vi "Autonomous Independent.vi"   [LabVIEW 2019]
doc: "This VI is called when autonomous begins, and will automatically be terminated when autonomous ends. You can carry out timed or sensor driven robot movement independently without needing to return to the caller."
uses:
  Robot Global Data.vi
  <vilib>/Rock Robotics/Network Tables/NT Read Number.vi
  <vilib>/Rock Robotics/Network Tables/NT Read String.vi
  <vilib>/Rock Robotics/Network Tables/NT Write Numeric Array.vi
panel:
  # "Be sure to right-click and choose Data Operations>>Make Current Value default if you want to save the array values with the VI"
types:
  T1 = typedef "WPI_JoystickDevRef.ctl" = cluster{"Device":T2}
  T2 = typedef "WPI_JoystickDeviceEnum.ctl" = enum16{"USB 0", "USB 1", "USB 2", "USB 3", "USB 4", "USB 5"}
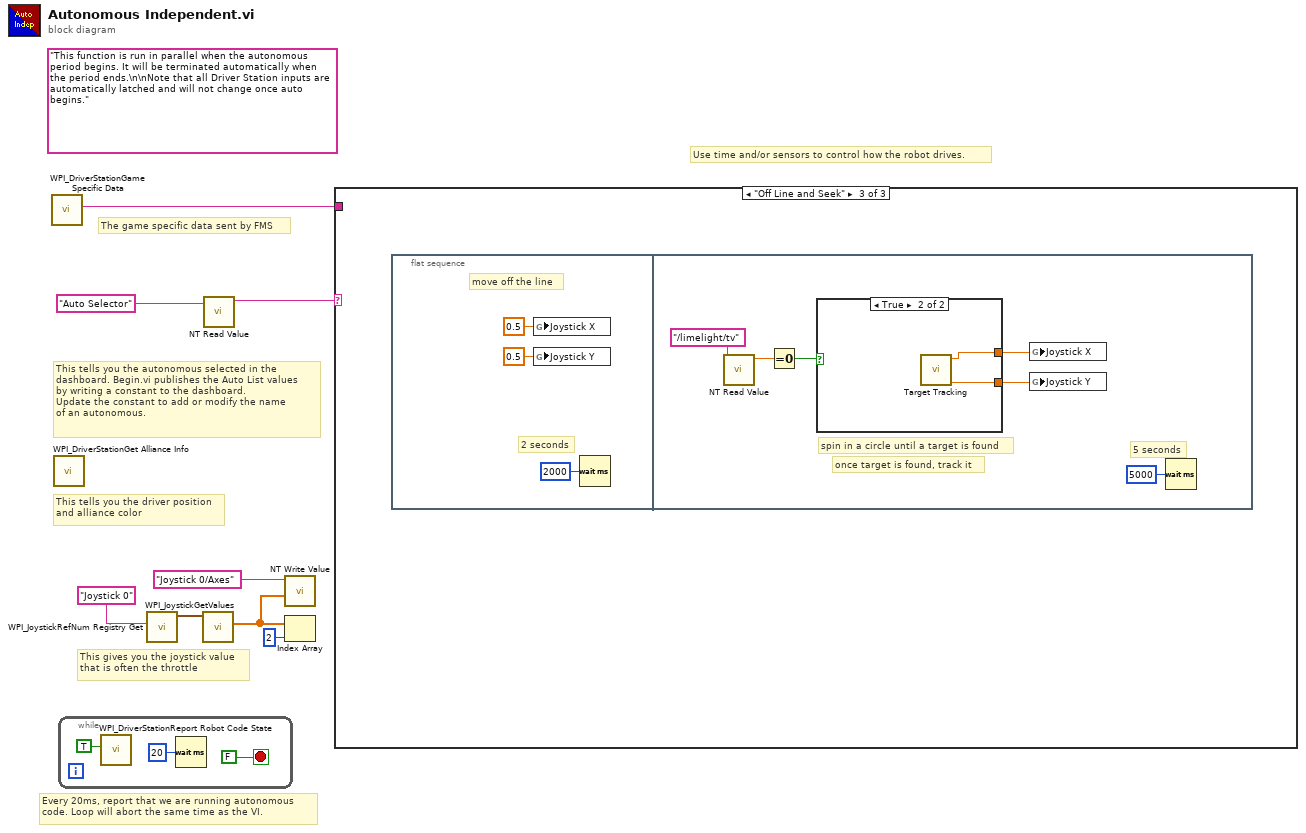
[diagram p0: block diagram]
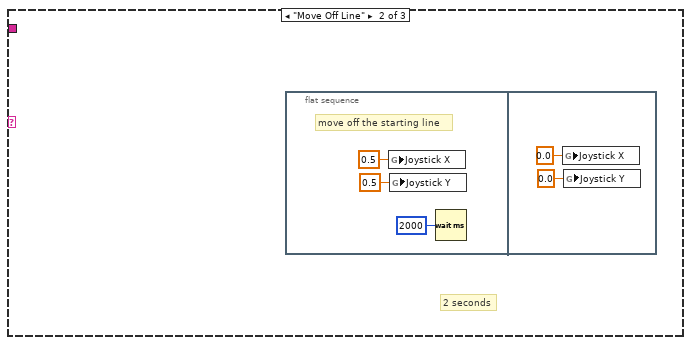
[diagram p3: hidden frame]
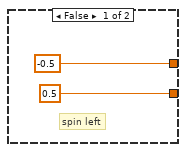
[diagram p4: hidden frame]
diagram:
  (unwired) "This function is run in parallel when the autonomous period begins. It will be terminated automatically when the period ends.\n\nNote that all Driver Station inputs are automatically latched and will not change once auto begins."
  # "The game specific data sent by FMS"
  # "This tells you the autonomous selected in the \ndashboard. Begin.vi publishes the Auto List values\nby writing a constant to the dashboard.\nUpdate the constant to add or modify the name\nof an autonomous."
  # "Every 20ms, report that we are running autonomous\ncode. Loop will abort the same time as the VI."
  # "This gives you the joystick value\nthat is often the throttle"
  # "Use time and/or sensors to control how the robot drives."
  # "This tells you the driver position\nand alliance color"
  n1 = call <vilib>:"WPI_DriverStationGame Specific Data.vi"() -> ("Game Specific Data"=w1:string)  [unwired: 11 in]
  n2 = call <vilib>:"WPI_DriverStationGet Alliance Info.vi"() -> ()  [unwired: 12 out]
  n3 = while {
    stop <- FALSE stop-if-true
    n4 = call <vilib>:"WPI_DriverStationReport Robot Code State.vi"("Autonomous"=TRUE) -> ()  [unwired: 10 in, 1 out]
    n5 = Wait (ms)(milliseconds to wait=u32 20) -> ()  [unwired: 1 out]
  }
  n6 = call <vilib>:"WPI_JoystickRefNum Registry Get.vi"("refnum name"="Joystick 0") -> ("JoystickDevRef"=w7:T1)  [unwired: 1 in, 9 out]
  n7 = call <vilib>:"WPI_JoystickGetValues.vi"("JoystickDevRef"=w7) -> ("Axes"=w3:dbl[])  [unwired: 6 in, 4 out]
  n8 = call-poly <vilib>:"NT Read Value.vi"("Name"="Auto Selector") -> ("String"=w4:string)  [unwired: 9 in, 1 out]
  n9 = call-poly <vilib>:"NT Write Value.vi"("Numeric Array"=w3, "Name"="Joystick 0/Axes") -> ()  [unwired: 9 in, 1 out]
  n10 = Index Array(array=w3, index=2) -> ()  [unwired: 1 out]
  n11 = case shown="\"Off Line and Seek\"" w4 {
    tunnel: w1 -> [_ _ _]
    frame Default {
      # "You can put your main auto here, or you can right-click on the case and make any\nother frame be the default case."
      # "This is the frame that will execute if no selection is made, or if it is not recognized"
    }
    frame "Move Off Line" {
      # "2 seconds"
      n12 = flat-sequence {
        frame #0 {
          # "move off the starting line"
          n13 = global write "Robot Global Data.vi" "Joystick X"(0.5 ("Joystick X")) -> ()
          n14 = global write "Robot Global Data.vi" "Joystick Y"(0.5 ("Joystick Y")) -> ()
          n15 = Wait (ms)(milliseconds to wait=u32 2000) -> ()  [unwired: 1 out]
        }
        frame #1 {
          n16 = global write "Robot Global Data.vi" "Joystick X"(0.0 ("Joystick X")) -> ()
          n17 = global write "Robot Global Data.vi" "Joystick Y"(0.0 ("Joystick Y")) -> ()
        }
      }
    }
    frame "Off Line and Seek" {
      n18 = flat-sequence {
        frame #0 {
          # "move off the line"
          # "2 seconds"
          n19 = global write "Robot Global Data.vi" "Joystick X"(0.5 ("Joystick X")) -> ()
          n20 = global write "Robot Global Data.vi" "Joystick Y"(0.5 ("Joystick Y")) -> ()
          n21 = Wait (ms)(milliseconds to wait=u32 2000) -> ()  [unwired: 1 out]
        }
        frame #1 {
          # "5 seconds"
          # "once target is found, track it"
          # "spin in a circle until a target is found"
          n22 = call-poly <vilib>:"NT Read Value.vi"("Name"="/limelight/tv") -> ("Numeric"=w23:dbl)  [unwired: 9 in, 1 out]
          n23 = Equal To 0?(x=w23) -> (x = 0?=w24:bool)
          n24 = case shown="True" w24 {
            tunnel: [0.5 ("Joystick Y") w28] -> w22
            tunnel: [-0.5 ("Joystick X") w29] -> w21
            frame False {
              # "spin left"
            }
            frame True {
              n25 = call "Target Tracking.vi"() -> ("Joystick Y"=w28:dbl, "Joystick X"=w29:dbl)  [unwired: 10 in]
            }
          }
          n26 = global write "Robot Global Data.vi" "Joystick X"(w21) -> ()
          n27 = global write "Robot Global Data.vi" "Joystick Y"(w22) -> ()
          n28 = Wait (ms)(milliseconds to wait=u32 5000) -> ()  [unwired: 1 out]
        }
      }
    }
  }
